vi "Add Experiment Description Comments.vi"(7 "error in (no error)":errorcluster, 9 "Experiment Description":string, 10 "Comments in":string) -> (0 "error out":errorcluster, 3 "Comments":string)   [LabVIEW 2016, in "Control Experiment.lvclass"]
uses:
  Control Experiment.lvclass
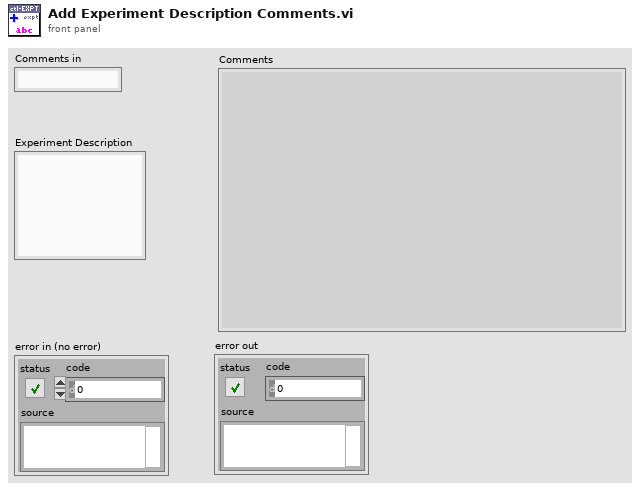
[diagram p1: front panel]
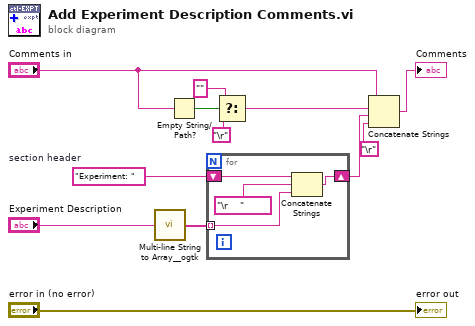
[diagram p0: block diagram]
diagram:
  w7 = "Experiment: "  # section header
  n1 = call <userlib>:"Multi-line String to Array__ogtk.vi"("string"="Experiment Description") -> ("lines"=w8:string[])
  n2 = Empty String/Path?(string/path="Comments in") -> (empty?=w11:bool)
  n3 = for {
    shift-right: [w16] -> w2
    shift-left: w7 -> [w15]
    tunnel: w8 -> [w13] mode=indexing
    n4 = Concatenate Strings(w15, "\r    " ("string"), w13) -> (w16:string)
  }
  n5 = Select(t="", s=w11, f="\r") -> (s? t:f=w4:string)
  n6 = Concatenate Strings("Comments in", w4, w2, "\r") -> (→"Comments":string)
  "error out" <- "error in (no error)"
